vi "extracted timestamp to ns.vi"(11 "Time Stamp":timestamp) -> (3 "nominal core ns":i64)   [LabVIEW 2026, in "Nominal Core Streaming Engine.lvlib"]
doc: "Hand-inlines code from the LabVIEW open source project, license retrieved 08 21 2026\nVIPM: Epoch Date and Time\nContributors: \nPatrick Irvin (@ciozi137)\nFrancois Normandin (@francois-normandin)\nJames Powell (@drjdpowell)\n\n\n\nZero-Clause BSD\nPermission to use, copy, modify, and/or distribute this software for any purpose with or without fee is hereby granted.\n\nTHE SOFTWARE IS PROVIDED \"AS IS\" AND THE AUTHOR DISCLAIMS ALL WARRANTIES WITH REGARD TO THIS SOFTWARE INCLUDING ALL IMPLIED\nWARRANTIES OF MERCHANTABILITY AND FITNESS. IN NO EVENT SHALL THE AUTHOR BE LIABLE FOR ANY SPECIAL, DIRECT, INDIRECT, OR\nCONSEQUENTIAL DAMAGES OR ANY DAMAGES WHATSOEVER RESULTING FROM LOSS OF USE, DATA OR PROFITS, WHETHER IN AN ACTION OF CONTRACT,\nNEGLIGENCE OR OTHER TORTIOUS ACTION, ARISING OUT OF OR IN CONNECTION WITH THE USE OR PERFORMANCE OF THIS SOFTWARE."
uses:
  Nominal Core Streaming Engine.lvlib
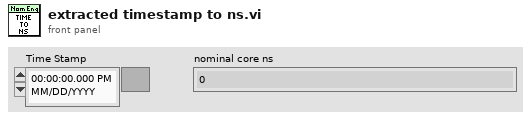
[diagram p1: front panel]
types:
  T1 = typedef "LVDateTimeRec.ctl" = cluster{"fractional second":dbl, "second":i32, "minute":i32, "hour":i32, "day of month":i32, "month":i32, "year":i32, "day of week":i32, "day of year":i32, "DST":i32}
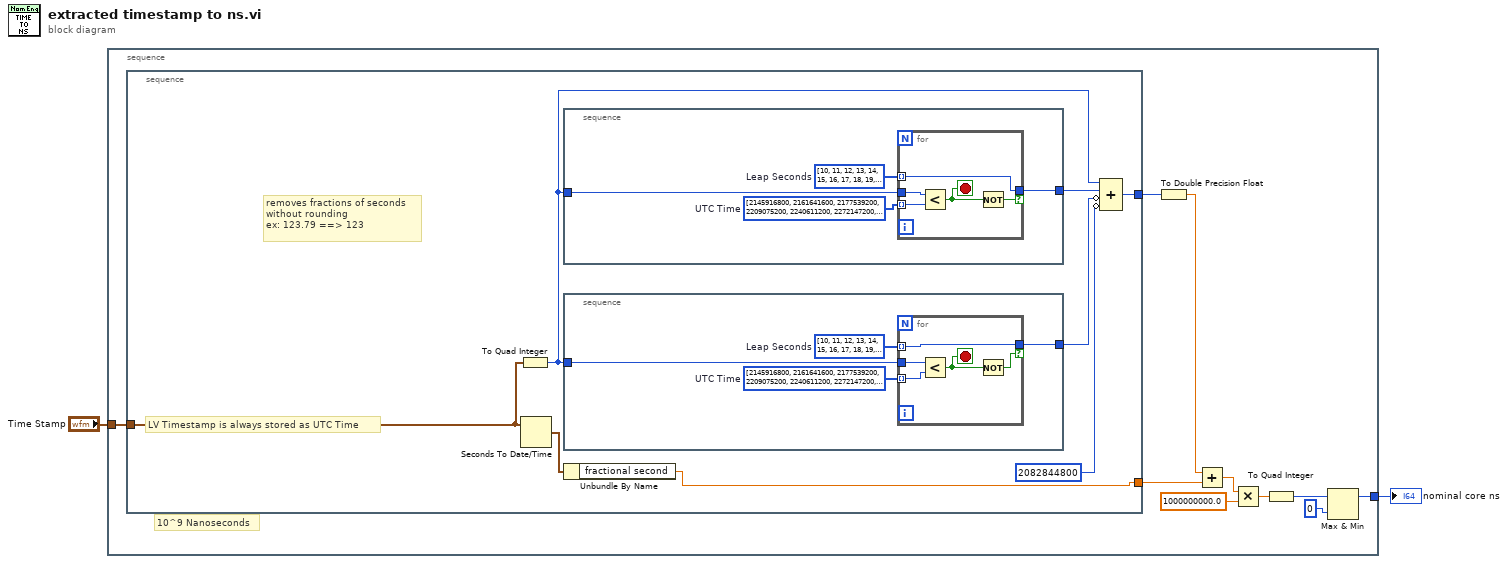
[diagram p0: block diagram]
diagram:
  n1 = stacked-sequence {
    tunnel: [w11] -> w2
    tunnel: "Time Stamp" -> [w12]
    frame #0 {
      # "10^9 Nanoseconds"
      n2 = stacked-sequence {
        tunnel: [w20] -> w5
        tunnel: [w15] -> w4
        tunnel: w12 -> [w14]
        frame #0 {
          # "LV Timestamp is always stored as UTC Time"
          # "removes fractions of seconds\nwithout rounding\nex: 123.79 ==> 123"
          n3 = To Quad Integer(1:w14) -> (0:w16:i64)
          n4 = Seconds To Date/Time(time stamp (now)=w14) -> (date time rec=w19:T1)  [unwired: 1 in]
          n5 = stacked-sequence {
            tunnel: [w33] -> w18
            tunnel: w16 -> [w31]
            frame #0 {
              w32 = i64[] [10, 11, 12, 13, 14, 15, 16, 17, 18, 19, 20, 21, 22, 23, 24, 25, 26, 27, 28, 29, 30, 31, 32, 33, 34, 35, 36, 37]  # Leap Seconds
              w30 = i64[] [2145916800, 2161641600, 2177539200, 2209075200, 2240611200, 2272147200, 2303769600, 2335305600, 2366841600, 2398377600, 2445638400, 2477174400, 2508710400, 2571868800, 2650838400, 2713996800, 2745532800, 2792793600, 2824329600, 2855865600, 2903299200, 2950560000, 2997993600, 3218918400, 3313612800, 3423945600, 3518553600, 3566073600]  # UTC Time
              n6 = for {
                tunnel: w30 -> [w38] mode=indexing
                tunnel: w31 -> [w37]
                tunnel: w32 -> [w36] mode=indexing
                tunnel: [w36] -> w33 if=w34
                stop <- w35 stop-if-true
                n7 = Less?(x=w37, y=w38) -> (x < y?=w35:bool)
                n8 = Not(x=w35) -> (.not. x?=w34:bool)
              }
            }
          }
          n9 = stacked-sequence {
            tunnel: [w24] -> w17
            tunnel: w16 -> [w23]
            frame #0 {
              w22 = i64[] [10, 11, 12, 13, 14, 15, 16, 17, 18, 19, 20, 21, 22, 23, 24, 25, 26, 27, 28, 29, 30, 31, 32, 33, 34, 35, 36, 37]  # Leap Seconds
              w21 = i64[] [2145916800, 2161641600, 2177539200, 2209075200, 2240611200, 2272147200, 2303769600, 2335305600, 2366841600, 2398377600, 2445638400, 2477174400, 2508710400, 2571868800, 2650838400, 2713996800, 2745532800, 2792793600, 2824329600, 2855865600, 2903299200, 2950560000, 2997993600, 3218918400, 3313612800, 3423945600, 3518553600, 3566073600]  # UTC Time
              n10 = for {
                tunnel: w21 -> [w29] mode=indexing
                tunnel: w23 -> [w28]
                tunnel: w22 -> [w27] mode=indexing
                tunnel: [w27] -> w24 if=w25
                stop <- w26 stop-if-true
                n11 = Less?(x=w28, y=w29) -> (x < y?=w26:bool)
                n12 = Not(x=w26) -> (.not. x?=w25:bool)
              }
            }
          }
          n13 = Unbundle By Name(w19) -> ("fractional second"=w20:dbl)
          n14 = Compound Arithmetic op=ADD(w16, w18, invert w17, invert i64 2082844800 ("Timestamp Offset")) -> (w15:i64)
        }
      }
      n15 = To Double Precision Float(number=w4) -> (double precision float=w8:dbl)
      n16 = Add(x=w8, y=w5) -> (x+y=w6:dbl)
      n17 = Multiply(x=w6, y=1000000000.0) -> (x*y=w7:dbl)
      n18 = To Quad Integer(1:w7) -> (0:w9:i64)
      n19 = Max & Min(x=w9, y=i64 0) -> (max(x,y)=w11:i64)  [unwired: 1 out]
    }
  }
  "nominal core ns" <- w2
